vi "configuration UI.vi"() -> ()   [LabVIEW 2013, in "Scan Engine editor node.lvclass"]
uses:
  Scan Engine editor node.lvclass
  <vilib>/NI/Configuration Framework/Node/NodeRef.ctl
  <vilib>/NI/Configuration Framework/Node/NISE_CEF_Node.lvclass
  <vilib>/NI/AMC/Message Queue.ctl
  <vilib>/NI/AMC/Message.ctl
  <vilib>/NI/Tools/Keyed Array/KeyedArray.ctl
  <vilib>/NI/Configuration Framework/Node/UserEventRef.ctl
  <vilib>/NI/Configuration Framework/Controls/EventCluster.ctl
  <vilib>/NI/DCAF UI Toolkit/Controls/Configure.ctl
  <vilib>/NI/DCAF UI Toolkit/Controls/Add.ctl
  <vilib>/NI/DCAF UI Toolkit/Controls/Remove.ctl
  <vilib>/NI/Configuration Framework/Node/StopEvent.ctl
  <vilib>/NI/Configuration Framework/Node/RefreshUIEvent.ctl
  <vilib>/NI/Configuration Framework/Node/CacheState.ctl
  <vilib>/NI/Configuration Framework/Node/NodeChangeEvent.ctl
  <vilib>/NI/Tag Bus/tag/Data Type.ctl
  Permissions Enum.ctl
  <vilib>/NI/DCAF/Tag Editor Core/control module/editor node/channel action event.ctl
  <vilib>/NI/DCAF/Tag Editor Core/control module/editor node/dialog output action.ctl
  <vilib>/NI/Tag Bus Module Framework/channel/TBM channel.lvclass
  <vilib>/NI/Tag Bus/tag/tag descriptor.lvclass
  <vilib>/NI/DCAF UI Toolkit/Controls/Import.ctl
  <vilib>/NI/DCAF/Tag Editor Core/Table API/Table Manager/references.ctl
  <vilib>/NI/DCAF/Tag Editor Core/Table API/Listbox/Multi Column Listbox.lvclass
  configuration/Scan Engine configuration.lvclass
  <vilib>/Utility/miscctls.llb/LVPositionTypeDef.ctl
  <vilib>/NI/Configuration Framework/NISE_CEF_TreeControl.lvlib
  <vilib>/NI/Tools/Keyed Array/Tools_KeyedArray.lvlib
  <vilib>/NI/AMC/AMC.lvlib
  <vilib>/NI/DCAF/Tag Editor Core/control module/editor node/control module editor.lvclass
  <vilib>/NI/DCAF/Tag Editor Core/Table API/Table Manager/Table Manager.lvclass
  <vilib>/NI/DCAF UI Toolkit/Controls/DCAF UI Elements.lvlib
panel:
  in  "user event out":refnum<user-event>
  in  "Permissions":T1
  in  "data type":T2
  in  "node change":T3
  in  "cache state":T4
  in  "refresh UI":T5
  in  "stop event":T6
  in  "Tab Control":enum32{"Scan Engine Settings"}(tab)
  in  "Remove Button":T7
  in  "Add Button":T8
  in  "Table":i32(listbox)=13
  in  "settings":T9
  in  "Scan Period (uSec)":u32
  in  "Discover Channels?":bool
  in  "Import":T10
  in  "Generate Tags":bool
  in  "user event":T11
  in  "main queue":T12
  in  "node ref":T13
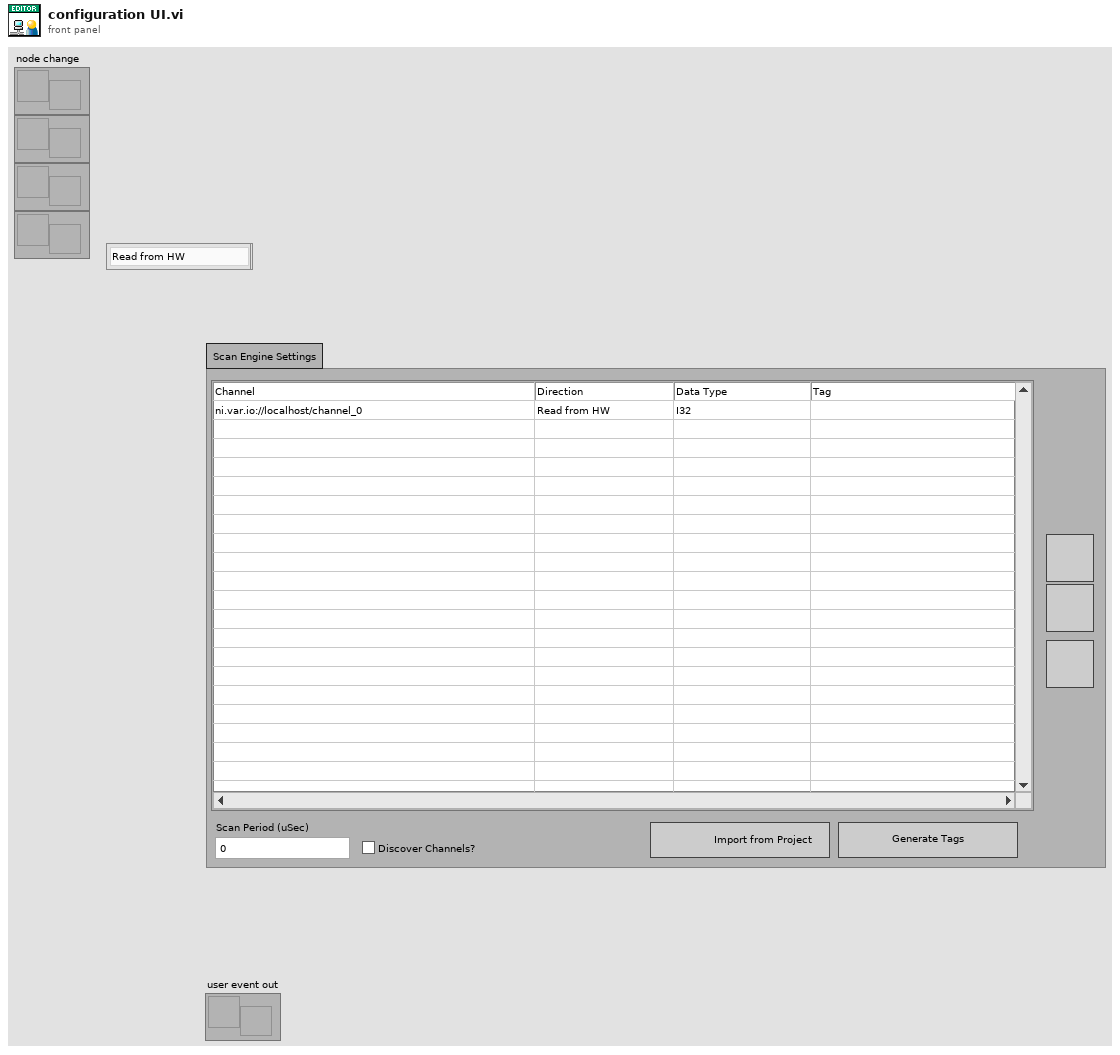
[diagram p1: front panel]
types:
  T1 = typedef "Scan Engine editor node.lvclass/Permissions Enum.ctl" = enum16{"Read from HW", "Write to HW"}
  T2 = typedef "tag bus.lvlib/tag descriptor.lvclass/Data Type.ctl" = enum16{"Double", "Single", "I64", "I32", "I16", "I8", "U64", "U32", "U16", "U8", "Boolean", "String", "Array of Double", "Array of Single", "Array of I64", "Array of I32", "Array of I16", "Array of I8", "Array of U64", "Array of U32", "Array of U16", "Array of U8", "Array of Boolean", "Array of String"}
  T3 = typedef "NISE_CEF_Node.lvclass/NodeChangeEvent.ctl" = refnum<user-event>
  T4 = typedef "NISE_CEF_Node.lvclass/CacheState.ctl" = refnum<user-event>
  T5 = typedef "NISE_CEF_Node.lvclass/RefreshUIEvent.ctl" = refnum<user-event>
  T6 = typedef "NISE_CEF_Node.lvclass/StopEvent.ctl" = refnum<user-event>
  T7 = typedef "DCAF UI Elements.lvlib/Remove.ctl" = bool
  T8 = typedef "DCAF UI Elements.lvlib/Add.ctl" = bool
  T9 = typedef "DCAF UI Elements.lvlib/Configure.ctl" = bool
  T10 = typedef "DCAF UI Elements.lvlib/Import.ctl" = bool
  T11 = typedef "NISE_CEF_Node.lvclass/UserEventRef.ctl" = refnum<user-event>
  T12 = typedef "AMC.lvlib/Message Queue.ctl" = refnum<queue>
  T13 = typedef "NISE_CEF_Node.lvclass/NodeRef.ctl" = refnum<data-value>
  T14 = typedef "Table Manager.lvlib/Table Manager.lvclass/references.ctl" = cluster{"stop event":T6, "refresh UI":T5, "cache state":T4, "node change":T3, "user event out":refnum<user-event>, "main queue":T12, "user event":T11}
  T15 = typedef "LVPositionTypeDef.ctl" = cluster{"Left":i32, "Top":i32}
  T16 = typedef "Table Manager.lvlib/Table Manager.lvclass/object ref.ctl" = cluster{"engine":refnum<data-value>, "Node Ref":refnum<data-value>}
  T17 = typedef "Table Manager.lvlib/Column.lvclass/Column Descriptor.ctl" = cluster{"name":string, "caption":string, "Column Type":T18, "Params":string, "AutoSizeMode":i32, "FillWeight":sgl, "MinWidth":u32, "tooltip":string, "Enum Reference":refnum<vi>, "Channel suffix":string, "Read Only":bool, "Call Back VI":T19, "DT Dependency":i32, "name dependency":i32, "data type":T2, "Custom Column":refnum<class "Column.lvclass">}
  T18 = typedef "Table Manager.lvlib/Column.lvclass/Column Type.ctl" = enum16{"String", "Mapping", "Enum", "Custom"}
  T19 = typedef "Table Manager.lvlib/Table Manager.lvclass/Call Back Ref Type Def.ctl" = refnum<vi>
  T20 = typedef "Table Manager.lvlib/Table Manager.lvclass/Table Events.ctl" = cluster{"Menu Selection":refnum<user-event>}
  T21 = enum8{"Enabled", "Disabled", "Disabled and Grayed Out"}
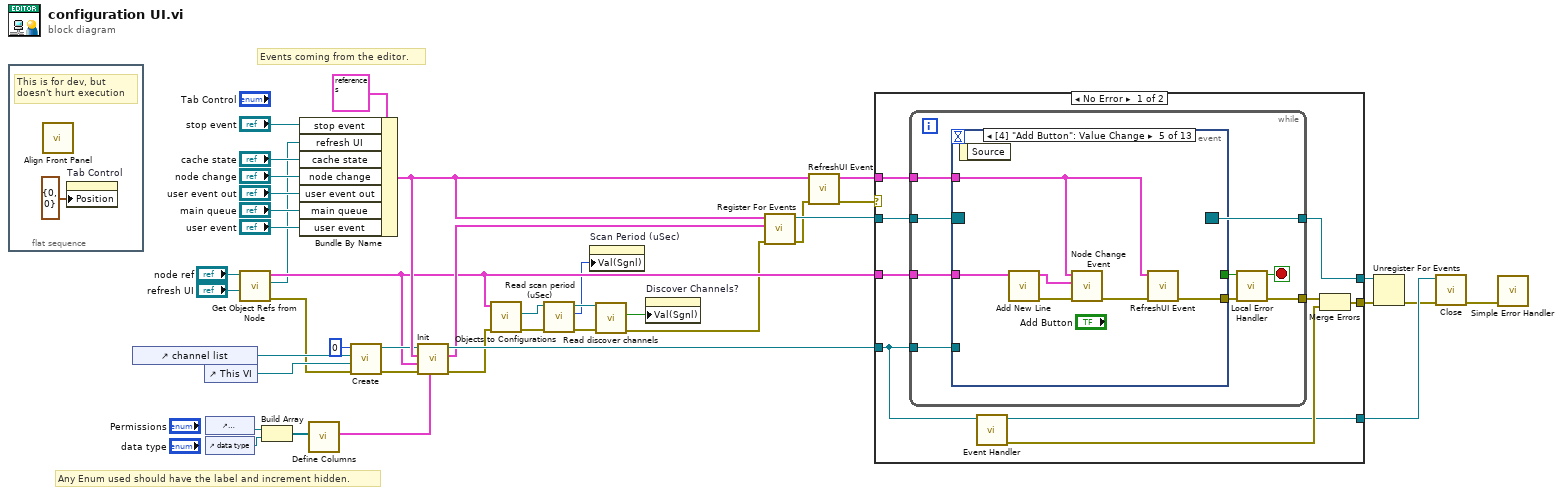
[diagram p0: block diagram]
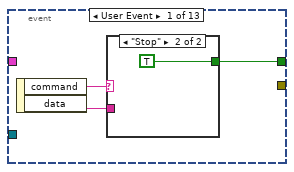
[diagram p2: hidden frame]
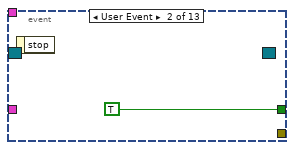
[diagram p4: hidden frame]
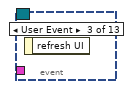
[diagram p5: hidden frame]
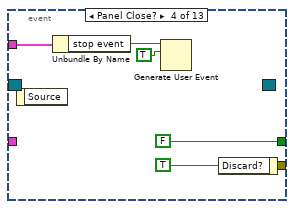
[diagram p6: hidden frame]
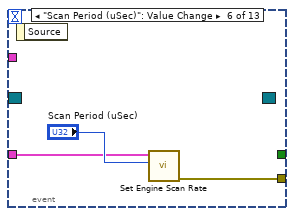
[diagram p7: hidden frame]
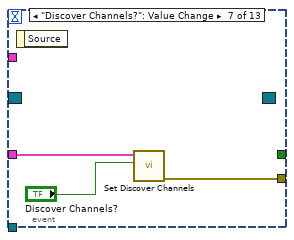
[diagram p8: hidden frame]
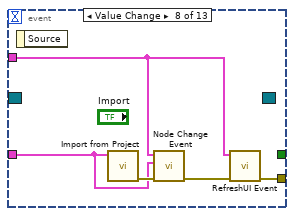
[diagram p9: hidden frame]
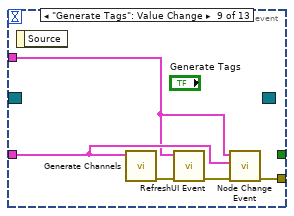
[diagram p10: hidden frame]
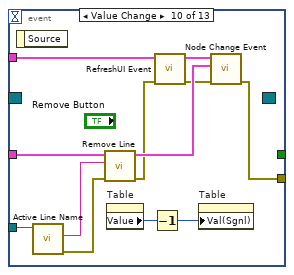
[diagram p11: hidden frame]
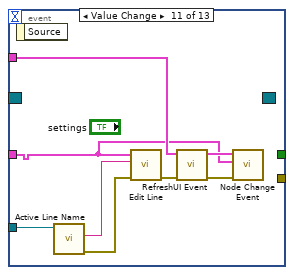
[diagram p12: hidden frame]
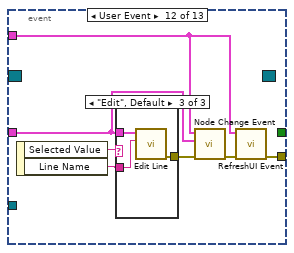
[diagram p13: hidden frame]
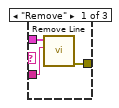
[diagram p14: hidden frame]
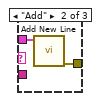
[diagram p15: hidden frame]
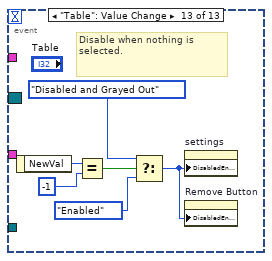
[diagram p16: hidden frame]
diagram:
  # "Any Enum used should have the label and increment hidden."
  # "Events coming from the editor."
  n1 = flat-sequence {
    frame #0 {
      # "This is for dev, but doesn't hurt execution"
      n2 = call <vilib>:"Align Front Panel.vi"() -> ()  [unwired: 10 in, 2 out]
      n3 = property on="Tab Control" class="TabCtl (strict)"("Position"=T15 {"Left"=0, "Top"=0}) -> ()  [unwired: 2 in, 2 out]
    }
  }
  n4 = control-ref of="channel list"() -> (w21:refnum<vi>)
  n5 = control-ref of="This VI"() -> (w19:refnum<vi>)
  n6 = control-ref of="Permissions"() -> (w28:refnum<vi>)
  n7 = control-ref of="data type"() -> (w27:refnum<vi>)
  n8 = call "Get Object Refs from Node.vi"("refresh UI"="refresh UI", "Data Value Reference in"="node ref") -> ("error out"=w3:errorcluster, "refresh UI out"=w4:T5, "references"=w15:T16)  [unwired: 7 in]
  n9 = Build Array(w28, w27) -> (w26:refnum<vi>[])
  n10 = Bundle By Name(cluster=T14 {"stop event"=refnum, "refresh UI"=refnum, "cache state"=refnum, "node change"=refnum, "user event out"=refnum, "main queue"=refnum, "user event"=refnum} ("References"), "stop event"="stop event", "refresh UI"=w4, "cache state"="cache state", "node change"="node change", "user event out"="user event out", "main queue"="main queue", "user event"="user event") -> (w29:T14)
  n11 = call "Define Columns.vi"("Enum Array"=w26) -> ("Column Definition"=w31:T17[])  [unwired: 10 in]
  n12 = call <vilib>:"Create.vi"("error in (no error)"=w3, "Top VI"=w19, "Listbox"=w21, "Index"=0) -> ("error out"=w2:errorcluster, "reference out"=w18:refnum<class "Multi Column Listbox.lvclass">)  [unwired: 6 in]
  n13 = call-dynamic "Init.vi"("Column Descriptors"=w31, "error in (no error)"=w2, "Node object refs"=w15, "Event References"=w29, "Multi Column Listbox in"=w18) -> ("error out"=w17:errorcluster, "Table Events"=w16:T20, "Multi Column Listbox out"=w25:refnum<class "Multi Column Listbox.lvclass">)  [unwired: 4 in]
  n14 = call "Objects to Configurations.vi"("error in (no error)"=w17, "Objects in"=w15) -> ("error out"=w11:errorcluster, "tag bus configurable plugin module configuration"=w14:refnum<class "Scan Engine configuration.lvclass">)  [unwired: 7 in, 1 out]
  n15 = call-dynamic "Read scan period (uSec).vi"("error in (no error)"=w11, "Scan Engine configuration1 in"=w14) -> ("error out"=w12:errorcluster, "scan period (uSec)"=w10:u32, "Scan Engine configuration1 out"=w13:refnum<class "Scan Engine configuration.lvclass">)  [unwired: 7 in]
  n16 = property on="Scan Period (uSec)" class="DigNum (strict)"("Val(Sgnl)"=w10) -> ()  [unwired: 2 in, 2 out]
  n17 = call-dynamic "Read discover channels.vi"("error in (no error)"=w12, "Scan Engine configuration1 in"=w13) -> ("error out"=w1:errorcluster, "discover channels"=w9:bool)  [unwired: 7 in, 1 out]
  n18 = property on="Discover Channels?" class="Bool (strict)"("Val(Sgnl)"=w9) -> ()  [unwired: 2 in, 2 out]
  n19 = call "Register For Events.vi"("error in"=w1, "Table Events"=w16, "References"=w29) -> ("error out"=w23:errorcluster, "Event Registration Refnum"=w32:refnum<event-registration>)  [unwired: 7 in]
  n20 = call "RefreshUI Event.vi"("error in (no error)"=w23, "References in"=w29) -> ("error out"=w22:errorcluster, "References out"=w30:T14)  [unwired: 8 in]
  n21 = case shown="No Error" w22 {
    selector: w22 -> [_ w134]
    tunnel: w32 -> [w51 w133]
    tunnel: [w50 w133] -> w41
    tunnel: [w44 w134] -> w40
    tunnel: w30 -> [w49 _]
    tunnel: w15 -> [w48 _]
    tunnel: w25 -> [w47 w132]
    tunnel: [w43 w132] -> w8
    frame No Error {
      n22 = while {
        tunnel: w51 -> [w60]
        tunnel: [w59] -> w50
        tunnel: [w56] -> w45
        tunnel: w49 -> [w54]
        tunnel: w48 -> [w53]
        tunnel: w47 -> [w52]
        stop <- w58 stop-if-true
        n23 = event shown="[4] \"Add Button\": Value Change" {
          selector: w60 -> [_ _ _ _ _ _ _ _ _ _ _ _ _]
          dyn-events: [_ _ _ _ _ _ _ _ _ _ _ _ _] -> w59
          timeout: _ -> [_ _ _ _ _ _ _ _ _ _ _ _ _]
          tunnel: [w63 TRUE _ FALSE _ _ _ _ _ _ _ _ _] -> w57
          tunnel: [_ _ _ _ w71 w76 w79 w84 w87 w97 _ w115 _] -> w55
          tunnel: w54 -> [_ _ _ w67 w74 _ _ w83 w88 w102 w105 w111 _]
          tunnel: w53 -> [_ _ _ _ w75 w77 w81 w82 w89 w101 w104 w112 _]
          tunnel: w52 -> [_ _ _ _ _ _ _ _ _ w96 w110 _ _]
          event User Event {
            n24 = event-data() -> ("command"=w62:string, "data"=w61:string)  [unwired: 1 in]
            n25 = case shown="\"Stop\"" w62 {
              tunnel: [_ TRUE] -> w63
              tunnel: w61 -> [_ _]
              frame Default {
              }
              frame "Stop" {
              }
            }
          }
          event User Event {
            n26 = event-data() -> ()  [unwired: 1 in, 1 out]
          }
          event User Event {
            n27 = event-data() -> ()  [unwired: 1 in, 1 out]
          }
          event Panel Close? {
            n28 = event-data() -> ()  [unwired: 1 in, 1 out]
            n29 = Unbundle By Name(w67) -> ("stop event"=w66:T6)
            n30 = Generate User Event(user event=w66, event data cluster=TRUE ("event data")) -> ()  [unwired: 2 in, 2 out]
            n31 = event-data("Discard?"=TRUE) -> ()  [unwired: 1 in, 1 out]
          }
          event Value Change {
            n32 = event-data() -> ()  [unwired: 1 in, 1 out]
            n33 = call "Add New Line.vi"("objects"=w75) -> ("error out"=w73:errorcluster)  [unwired: 9 in, 1 out]
            n34 = call "Node Change Event.vi"("error in (no error)"=w73, "objects"=w75, "References in"=w74) -> ("error out"=w72:errorcluster)  [unwired: 8 in]
            n35 = call "RefreshUI Event.vi"("error in (no error)"=w72, "References in"=w74) -> ("error out"=w71:errorcluster)  [unwired: 8 in, 1 out]
          }
          event "Scan Period (uSec)": Value Change {
            n36 = event-data() -> ()  [unwired: 1 in, 1 out]
            n37 = call "Set Engine Scan Rate.vi"("scan period (uSec)"="Scan Period (uSec)", "references in"=w77) -> ("error out"=w76:errorcluster)  [unwired: 8 in, 1 out]
          }
          event "Discover Channels?": Value Change {
            n38 = event-data() -> ()  [unwired: 1 in, 1 out]
            n39 = call "Set Discover Channels.vi"("discover channels"="Discover Channels?", "references in"=w81) -> ("error out"=w79:errorcluster)  [unwired: 8 in, 1 out]
          }
          event Value Change {
            n40 = event-data() -> ()  [unwired: 1 in, 1 out]
            n41 = call "Import from Project.vi"("references"=w82) -> ("error out"=w86:errorcluster)  [unwired: 9 in, 1 out]
            n42 = call "Node Change Event.vi"("error in (no error)"=w86, "objects"=w82, "References in"=w83) -> ("error out"=w85:errorcluster)  [unwired: 8 in]
            n43 = call "RefreshUI Event.vi"("error in (no error)"=w85, "References in"=w83) -> ("error out"=w84:errorcluster)  [unwired: 8 in, 1 out]
          }
          event "Generate Tags": Value Change {
            n44 = event-data() -> ()  [unwired: 1 in, 1 out]
            n45 = call "Generate Channels.vi"("references in"=w89) -> ("error out"=w90:errorcluster)  [unwired: 10 in]
            n46 = call "RefreshUI Event.vi"("error in (no error)"=w90, "References in"=w88) -> ("error out"=w91:errorcluster)  [unwired: 8 in, 1 out]
            n47 = call "Node Change Event.vi"("error in (no error)"=w91, "objects"=w89, "References in"=w88) -> ("error out"=w87:errorcluster)  [unwired: 8 in]
          }
          event Value Change {
            n48 = event-data() -> ()  [unwired: 1 in, 1 out]
            n49 = call-dynamic "Active Line Name.vi"("Multi Column Listbox in"=w96) -> ("error out"=w94:errorcluster, "Active Line Name"=w95:string)  [unwired: 8 in, 1 out]
            n50 = call "Remove Line.vi"("error in"=w94, "Active Line Name"=w95, "Objects"=w101) -> ("error out"=w98:errorcluster)  [unwired: 8 in]
            n51 = property on="Table" class="MCListbox (strict)"() -> ("Value"=w93:i32)  [unwired: 2 in, 2 out]
            n52 = Decrement(x=w93) -> (x-1=w92:i32)
            n53 = call "RefreshUI Event.vi"("error in (no error)"=w98, "References in"=w102) -> ("error out"=w100:errorcluster, "References out"=w99:T14)  [unwired: 8 in]
            n54 = property on="Table" class="MCListbox (strict)"("Val(Sgnl)"=w92) -> ()  [unwired: 2 in, 2 out]
            n55 = call "Node Change Event.vi"("error in (no error)"=w100, "objects"=w101, "References in"=w99) -> ("error out"=w97:errorcluster)  [unwired: 8 in]
          }
          event Value Change {
            n56 = event-data() -> ()  [unwired: 1 in, 1 out]
            n57 = call-dynamic "Active Line Name.vi"("Multi Column Listbox in"=w110) -> ("error out"=w108:errorcluster, "Active Line Name"=w109:string)  [unwired: 8 in, 1 out]
            n58 = call "Edit Line.vi"("error in"=w108, "Line Name"=w109, "References"=w104) -> ("error out"=w103:errorcluster)  [unwired: 7 in, 1 out]
            n59 = call "RefreshUI Event.vi"("error in (no error)"=w103, "References in"=w105) -> ("error out"=w106:errorcluster, "References out"=w107:T14)  [unwired: 8 in]
            n60 = call "Node Change Event.vi"("error in (no error)"=w106, "objects"=w104, "References in"=w107) -> ()  [unwired: 8 in, 1 out]
          }
          event User Event {
            n61 = event-data() -> ("Selected Value"=w117:string, "Line Name"=w114:string)  [unwired: 1 in]
            n62 = case shown="\"Edit\", Default" w117 {
              tunnel: w114 -> [w120 _ w125]
              tunnel: w112 -> [w119 w122 w124]
              tunnel: [w118 w121 w123] -> w113
              frame "Remove" {
                n63 = call "Remove Line.vi"("Active Line Name"=w120, "Objects"=w119) -> ("error out"=w118:errorcluster)  [unwired: 9 in]
              }
              frame "Add" {
                n64 = call "Add New Line.vi"("objects"=w122) -> ("error out"=w121:errorcluster)  [unwired: 9 in, 1 out]
              }
              frame "Edit", Default {
                n65 = call "Edit Line.vi"("Line Name"=w125, "References"=w124) -> ("error out"=w123:errorcluster)  [unwired: 8 in, 1 out]
              }
            }
            n66 = call "Node Change Event.vi"("error in (no error)"=w113, "objects"=w112, "References in"=w111) -> ("error out"=w116:errorcluster)  [unwired: 8 in]
            n67 = call "RefreshUI Event.vi"("error in (no error)"=w116, "References in"=w111) -> ("error out"=w115:errorcluster)  [unwired: 8 in, 1 out]
          }
          event "Table": Value Change {
            # "Disable when nothing is selected."
            n68 = event-data() -> ("NewVal"=w131:i32)  [unwired: 1 in]
            n69 = Equal?(x=w131, y=-1) -> (x = y?=w129:bool)
            n70 = Select(t=T21."Disabled and Grayed Out" ("Disabled"), s=w129, f=T21."Enabled" ("Disabled")) -> (s? t:f=w127:T21)
            n71 = property on="settings" class="Bool"("DisabledEnum"=w127) -> ()  [unwired: 2 in, 2 out]
            n72 = property on="Remove Button" class="Bool"("DisabledEnum"=w127) -> ()  [unwired: 2 in, 2 out]
          }
        }
        n73 = call "Local Error Handler.vi"("error in"=w55, "Stop in"=w57) -> ("error out"=w56:errorcluster, "Stop out"=w58:bool)  [unwired: 8 in]
      }
      n74 = call-dynamic "Event Handler.vi"("Listbox in"=w47) -> ("error out"=w46:errorcluster, "Listbox out"=w43:refnum<class "Multi Column Listbox.lvclass">)  [unwired: 9 in]
      n75 = Merge Errors(w45, w46) -> (w44:errorcluster)
    }
    frame Error {
    }
  }
  n76 = Unregister For Events(event registration refnum=w41, error in=w40) -> (error out=w7:errorcluster)
  n77 = call-dynamic "Close.vi"("error in (no error)"=w7, "Multi Column Listbox in"=w8) -> ("error out"=w6:errorcluster)  [unwired: 8 in, 1 out]
  n78 = call <vilib>:"Simple Error Handler.vi"("error in (no error)"=w6) -> ()  [unwired: 4 in, 5 out]
